vi "test_F9P.vi"() -> ()   [LabVIEW 2019] (continued)
47,33,72,237,38,1*7F\r\n$GBGSV,4,4,13,34,13,141,,1*45\r\n$GBGSV,4,1,13,04,35,133,,05,09,257,,06,27,182,,07,09,201,,3*79\r\n$GBGSV,4,2,13,08,65,355,39,09,07,194,,10,16,222,16,11,38,142,21,3*7C\r\n$GBGSV,4,3,13,13,50,314,29,14,77,038,38,28,58,310,,33,72,237,,3*78\r\n$GBGSV,4,4,13,34,13,141,,3*47\r\n$GNGLL,3723.59889,N,12656.92573,E,064143.00,A,A*7F\r\n$GNRMC,064144.00,A,3723.59887,N,12656.92567,E,0.152,,250720,,,A,V*14\r\n$GNVTG,,T,,M,0.152,N,0.282,K,A*33\r\n$GNGGA,064144.00,3723.59887,N,12656.92567,E,1,12,0.77,63.9,M,18.5,M,,*75\r\n$GNGSA,A,3,17,19,06,05,02,12,09,,,,,,1.38,0.77,1.14,1*0A\r\n$GNGSA,A,3,85,70,71,72,,,,,,,,,1.38,0.77,1.14,2*05\r\n$GNGSA,A,3,36,11,04,09,12,,,,,,,,1.38,0.77,1.14,3*06\r\n$GNGSA,A,3,28,14,13,11,33,08,10,,,,,,1.38,0.77,1.14,4*0E\r\n$GPGSV,4,1,13,02,65,334,43,04,09,037,,05,47,260,41,06,59,075,34,1*60\r\n$GPGSV,4,2,13,07,06,105,,09,39,058,37,12,18,264,29,13,07,191,,1*62\r\n$GPGSV,4,3,13,17,20,157,22,19,38,161,34,25,11,294,,29,06,323,17,1*65\r\n$GPGSV,4,4,13,30,01,134,,1*52\r\n$GPGSV,4,1,13,02,65,334,,04,09,037,,05,47,260,30,06,59,075,21,6*62\r\n$GPGSV,4,2,13,07,06,105,,09,39,058,35,12,18,264,,13,07,191,,6*6C\r\n$GPGSV,4,3,13,17,20,157,,19,38,161,,25,11,294,,29,06,323,,6*63\r\n$GPGSV,4,4,13,30,01,134,,6*55\r\n$GLGSV,2,1,06,70,55,030,33,71,68,223,35,72,17,216,31,84,09,133,10,1*75\r\n$GLGSV,2,2,06,85,63,111,31,86,51,337,,1*78\r\n$GLGSV,2,1,06,70,55,030,,71,68,223,32,72,17,216,22,84,09,133,12,3*70\r\n$GLGSV,2,2,06,85,63,111,35,86,51,337,,3*7E\r\n$GAGSV,3,1,09,02,04,288,08,04,68,087,34,09,44,196,27,11,77,034,37,7*77\r\n$GAGSV,3,2,09,12,32,114,29,18,55,286,45,19,18,042,06,25,01,241,,7*72\r\n$GAGSV,3,3,09,36,34,314,25,7*49\r\n$GAGSV,3,1,09,02,04,288,,04,68,087,33,09,44,196,30,11,77,034,31,2*7D\r\n$GAGSV,3,2,09,12,32,114,15,18,55,286,42,19,18,042,,25,01,241,,2*79\r\n$GAGSV,3,3,09,36,34,314,23,2*4A\r\n$GBGSV,4,1,13,04,35,133,,05,09,257,,06,27,182,,07,09,201,,1*7B\r\n$GBGSV,4,2,13,08,65,355,38,09,07,194,,10,16,222,,11,38,142,24,1*7D\r\n$GBGSV,4,3,13,13,50,314,29,14,77,038,39,28,58,310,46,33,72,237,40,1*7D\r\n$GBGSV,4,4,13,34,13,141,,1*45\r\n$GBGSV,4,1,13,04,35,133,,05,09,257,,06,27,182,,07,09,201,,3*79\r\n$GBGSV,4,2,13,08,65,355,39,09,07,194,,10,16,222,18,11,38,142,33,3*71\r\n$GBGSV,4,3,13,13,50,314,31,14,77,038,38,28,58,310,,33,72,237,,3*71\r\n$GBGSV,4,4,13,34,13,141,,3*47\r\n$GNGLL,3723.59887,N,12656.92567,E,064144.00,A,A*73\r\n$GNRMC,064145.00,A,3723.59896,N,12656.92569,E,0.478,305.82,250720,,,A,V*04\r\n$GNVTG,305.82,T,,M,0.478,N,0.885,K,A*21\r\n$GNGGA,064145.00,3723.59896,N,12656.92569,E,1,12,0.62,63.6,M,18.5,M,,*71\r\n$GNGSA,A,3,17,19,06,05,02,12,09,,,,,,1.08,0.62,0.88,1*09\r\n$GNGSA,A,3,85,70,71,72,,,,,,,,,1.08,0.62,0.88,2*06\r\n$GNGSA,A,3,36,19,11,04,09,12,,,,,,,1.08,0.62,0.88,3*0D\r\n$GNGSA,A,3,28,14,13,11,33,08,10,,,,,,1.08,0.62,0.88,4*0D\r\n$GPGSV,4,1,13,02,65,334,43,04,09,037,24,05,47,260,40,06,59,075,36,1*65\r\n$GPGSV,4,2,13,07,06,105,,09,39,058,39,12,18,264,28,13,07,191,,1*6D\r\n$GPGSV,4,3,13,17,20,157,23,19,38,161,29,25,11,294,,29,06,323,15,1*6A\r\n$GPGSV,4,4,13,30,01,134,,1*52\r\n$GPGSV,4,1,13,02,65,334,,04,09,037,19,05,47,260,35,06,59,075,33,6*6C\r\n$GPGSV,4,2,13,07,06,105,,09,39,058,38,12,18,264,,13,07,191,,6*61\r\n$GPGSV,4,3,13,17,20,157,22,19,38,161,,25,11,294,,29,06,323,,6*63\r\n$GPGSV,4,4,13,30,01,134,,6*55\r\n$GLGSV,2,1,06,70,55,030,28,71,68,223,39,72,17,216,26,84,09,133,10,1*75\r\n$GLGSV,2,2,06,85,63,111,30,86,51,337,,1*79\r\n$GLGSV,2,1,06,70,55,030,,71,68,223,32,72,17,216,22,84,09,133,11,3*73\r\n$GLGSV,2,2,06,85,63,111,30,86,51,337,,3*7B\r\n$GAGSV,3,1,09,02,04,288,08,04,68,087,36,09,44,196,35,11,77,034,39,7*78\r\n$GAGSV,3,2,09,12,32,114,28,18,55,286,47,19,18,042,11,25,01,241,,7*77\r\n$GAGSV,3,3,09,36,34,314,31,7*4C\r\n$GAGSV,3,1,09,02,04,288,,04,68,087,33,09,44,196,29,11,77,034,33,2*77\r\n$GAGSV,3,2,09,12,32,114,19,18,55,286,43,19,18,042,,25,01,241,,2*74\r\n$GAGSV,3,3,09,36,34,314,24,2*4D\r\n$GBGSV,4,1,13,04,35,133,,05,09,257,,06,27,182,,07,09,201,,1*7B\r\n$GBGSV,4,2,13,08,65,355,39,09,07,194,,10,16,222,,11,38,142,22,1*7A\r\n$GBGSV,4,3,13,13,50,314,29,14,77,038,41,28,58,310,44,33,72,237,39,1*7E\r\n$GBGSV,4,4,13,34,13,141,,1*45\r\n$GBGSV,4,1,13,04,35,133,,05,09,257,,06,27,182,,07,09,201,,3*79\r\n$GBGSV,4,2,13,08,65,355,36,09,07,194,,10,16,222,17,11,38,142,31,3*73\r\n$GBGSV,4,3,13,13,50,314,31,14,77,038,35,28,58,310,,33,72,237,,3*7C\r\n$GBGSV,4,4,13,34,13,141,,3*47\r\n$GNGLL,3723.59896,N,12656.92569,E,064145.00,A,A*7C\r\n$GNRMC,064146.00,A,3723.59920,N,12656.92613,E,1.922,48.63,250720,,,A,V*33\r\n$GNVTG,48.63,T,,M,1.922,N,3.560,K,A*12\r\n$GNGGA,064146.00,3723.59920,N,12656.92613,E,1,12,0.65,62.9,M,18.5,M,,*79\r\n$GNGSA,A,3,17,19,06,05,02,12,09,,,,,,1.13,0.65,0.92,1*0F\r\n$GNGSA,A,3,85,70,71,72,,,,,,,,,1.13,0.65,0.92,2*00\r\n$GNGSA,A,3,36,19,11,04,09,12,,,,,,,1.13,0.65,0.92,3*0B\r\n$GNGSA,A,3,28,14,13,11,33,08,10,,,,,,1.13,0.65,0.92,4*0B\r\n$GPGSV,4,1,13,02,65,334,39,04,08,037,22,05,47,260,35,06,59,075,43,1*6F\r\n$GPGSV,4,2,13,07,06,105,,09,39,058,40,12,18,264,20,13,07,191,,1*6B\r\n$GPGSV,4,3,13,17,20,157,22,19,38,161,33,25,11,294,,29,06,323,14,1*61\r\n$GPGSV,4,4,13,30,01,134,,1*52\r\n$GPGSV,4,1,13,02,65,334,,04,08,037,18,05,47,260,34,06,59,075,29,6*66\r\n$GPGSV,4,2,13,07,06,105,,09,39,058,38,12,18,264,23,13,07,191,,6*60\r\n$GPGSV,4,3,13,17,20,157,20,19,38,161,,25,11,294,,29,06,323,,6*61\r\n$GPGSV,4,4,13,30,01,134,,6*55\r\n$GLGSV,2,1,06,70,55,030,28,71,68,223,33,72,17,216,24,84,09,133,08,1*74\r\n$GLGSV,2,2,06,85,63,111,24,86,51,337,,1*7C\r\n$GLGSV,2,1,06,70,55,030,,71,68,223,32,72,17,216,21,84,09,133,09,3*79\r\n$GLGSV,2,2,06,85,63,111,25,86,51,337,,3*7F\r\n$GAGSV,3,1,09,02,04,288,09,04,68,087,32,09,44,196,31,11,77,034,39,7*79\r\n$GAGSV,3,2,09,12,32,114,28,18,55,286,43,19,18,042,16,25,01,241,,7*74\r\n$GAGSV,3,3,09,36,34,314,25,7*49\r\n$GAGSV,3,1,09,02,04,288,,04,68,087,37,09,44,196,29,11,77,034,30,2*70\r\n$GAGSV,3,2,09,12,32,114,25,18,55,286,37,19,18,042,,25,01,241,,2*78\r\n$GAGSV,3,3,09,36,34,314,22,2*4B\r\n$GBGSV,4,1,13,04,35,133,,05,09,257,,06,27,182,,07,09,201,,1*7B\r\n$GBGSV,4,2,13,08,65,355,42,09,07,194,,10,16,222,,11,38,142,23,1*77\r\n$GBGSV,4,3,13,13,50,314,29,14,77,038,42,28,58,310,44,33,72,237,38,1*7C\r\n$GBGSV,4,4,13,34,13,141,,1*45\r\n$GBGSV,4,1,13,04,35,133,,05,09,257,,06,27,182,,07,09,201,,3*79\r\n$GBGSV,4,2,13,08,65,355,36,09,07,194,,10,16,222,18,11,38,142,27,3*7B\r\n$GBGSV,4,3,13,13,50,314,28,14,77,038,34,28,58,310,,33,72,237,,3*75\r\n$GBGSV,4,4,13,34,13,141,,3*47\r\n$GNGLL,3723.59920,N,12656.92613,E,064146.00,A,A*7D\r\n$GNRMC,064147.00,A,3723.59950,N,12656.92680,E,2.195,54.45,250720,,,A,V*31\r\n$GNVTG,54.45,T,,M,2.195,N,4.064,K,A*1A\r\n$GNGGA,064147.00,3723.59950,N,12656.92680,E,1,12,0.67,62.1,M,18.5,M,,*7F\r\n$GNGSA,A,3,17,19,06,05,02,12,09,,,,,,1.15,0.67,0.93,1*0A\r\n$GNGSA,A,3,85,70,71,72,,,,,,,,,1.15,0.67,0.93,2*05\r\n$GNGSA,A,3,36,19,11,04,09,12,,,,,,,1.15,0.67,0.93,3*0E\r\n$GNGSA,A,3,28,14,13,11,33,08,10,,,,,,1.15,0.67,0.93,4*0E\r\n$GPGSV,4,1,13,02,65,334,42,04,08,037,22,05,48,261,29,06,59,075,43,1*60\r\n$GPGSV,4,2,13,07,06,105,,09,39,058,40,12,18,264,21,13,07,191,,1*6A\r\n$GPGSV,4,3,13,17,20,157,22,19,38,161,29,25,11,294,,29,06,323,11,1*6F\r\n$GPGSV,4,4,13,30,01,134,,1*52\r\n$GPGSV,4,1,13,02,65,334,,04,08,037,18,05,48,261,34,06,59,075,40,6*67\r\n$GPGSV,4,2,13,07,06,105,,09,39,058,40,12,18,264,23,13,07,191,,6*6F\r\n$GPGSV,4,3,13,17,20,157,18,19,38,161,,25,11,294,,29,06,323,,6*6A\r\n$GPGSV,4,4,13,30,01,134,,6*55\r\n$GLGSV,2,1,06,70,55,030,28,71,68,223,39,72,17,216,26,84,09,133,08,1*7C\r\n$GLGSV,2,2,06,85,63,111,31,86,51,337,,1*78\r\n$GLGSV,2,1,06,70,55,030,,71,68,223,32,72,17,216,21,84,09,133,13,3*72\r\n$GLGSV,2,2,06,85,63,111,28,86,51,337,,3*72\r\n$GAGSV,3,1,09,02,04,288,09,04,68,087,42,09,44,196,25,11,77,034,39,7*7B\r\n$GAGSV,3,2,09,12,32,114,20,18,55,286,43,19,18,042,20,25,01,241,,7*79\r\n$GAGSV,3,3,09,36,34,314,26,7*4A\r\n$GAGSV,3,1,09,02,04,288,,04,68,087,40,09,44,196,23,11,77,034,31,2*7B\r\n$GAGSV,3,2,09,12,32,114,23,18,55,286,39,19,18,042,,25,01,241,,2*70\r\n$GAGSV,3,3,09,36,34,314,18,2*42\r\n$GBGSV,4,1,13,04,35,133,,05,09,257,,06,27,182,,07,09,201,,1*7B\r\n$GBGSV,4,2,13,08,65,355,38,09,07,194,,10,16,222,,11,38,142,22,1*7B\r\n$GBGSV,4,3,13,13,50,314,23,14,77,038,43,28,58,310,38,33,72,237,40,1*73\r\n$GBGSV,4,4,13,34,13,141,,1*45\r\n$GBGSV,4,1,13,04,35,133,,05,09,257,,06,27,182,,07,09,201,,3*79\r\n$GBGSV,4,2,13,08,65,355,36,09,07,194,,10,16,222,19,11,38,142,27,3*7A\r\n$GBGSV,4,3,13,13,50,314,26,14,77,038,39,28,58,310,,33,72,237,,3*76\r\n$GBGSV,4,4,13,34,13,141,,3*47\r\n$GNGLL,3723.59950,N,12656.92680,E,064147.00,A,A*71\r\n$GNRMC,064148.00,A,3723.59985,N,12656.92753,E,2.416,59.10,250720,,,A,V*3A\r\n$GNVTG,59.10,T,,M,2.416,N,4.474,K,A*1C\r\n$GNGGA,064148.00,3723.59985,N,12656.92753,E,1,12,0.62,61.5,M,18.5,M,,*75\r\n$GNGSA,A,3,17,19,06,05,02,12,09,,,,,,1.08,0.62,0.88,1*09\r\n$GNGSA,A,3,85,70,71,72,,,,,,,,,1.08,0.62,0.88,2*06\r\n$GNGSA,A,3,36,19,11,04,09,12,,,,,,,1.08,0.62,0.88,3*0D\r\n$GNGSA,A,3,28,14,13,11,33,08,10,,,,,,1.08,0.62,0.88,4*0D\r\n$GPGSV,4,1,13,02,65,334,46,04,08,037,21,05,48,261,38,06,58,076,44,1*62\r\n$GPGSV,4,2,13,07,06,105,,09,39,058,41,12,18,264,20,13,07,191,,1*6A\r\n$GPGSV,4,3,13,17,20,157,22,19,38,161,29,25,11,294,,29,06,323,,1*6F\r\n$GPGSV,4,4,13,30,01,134,,1*52\r\n$GPGSV,4,1,13,02,65,334,,04,08,037,29,05,48,261,34,06,58,076,36,6*66\r\n$GPGSV,4,2,13,07,06,105,,09,39,058,42,12,18,264,22,13,07,191,,6*6C\r\n$GPGSV,4,3,13,17,20,157,17,19,38,161,,25,11,294,,29,06,323,,6*65\r\n$GPGSV,4,4,13,30,01,134,,6*55\r\n$GLGSV,2,1,06,70,55,030,34,71,68,223,40,72,17,216,26,84,09,133,09,1*7E\r\n$GLGSV,2,2,06,85,63,111,31,86,51,337,,1*78\r\n$GLGSV,2,1,06,70,55,030,,71,68,223,27,72,17,216,19,84,09,133,08,3*77\r\n$GLGSV,2,2,06,85,63,111,27,86,51,337,,3*7D\r\n$GAGSV,3,1,09,02,04,288,10,04,68,087,42,09,44,196,30,11,77,034,39,7*77\r\n$GAGSV,3,2,09,12,32,114,22,18,55,286,44,19,18,042,20,25,01,241,,7*7C\r\n$GAGSV,3,3,09,36,34,314,25,7*49\r\n$GAGSV,3,1,09,02,04,288,,04,68,087,33,09,44,196,25,11,77,034,32,2*7A\r\n$GAGSV,3,2,09,12,32,114,26,18,55,286,43,19,18,042,,25,01,241,,2*78\r\n$GAGSV,3,3,09,36,34,314,19,2*43\r\n$GBGSV,4,1,13,04,35,133,,05,09,257,,06,27,182,,07,09,201,,1*7B\r\n$GBGSV,4,2,13,08,65,355,42,09,07,194,,10,16,222,,11,38,142,25,1*71\r\n$GBGSV,4,3,13,13,50,314,25,14,77,038,41,28,58,310,31,33,72,237,41,1*7F\r\n$GBGSV,4,4,13,34,13,141,,1*45\r\n$GBGSV,4,1,13,04,35,133,,05,09,257,,06,27,182,,07,09,201,,3*79\r\n$GBGSV,4,2,13,08,65,355,29,09,07,194,,10,16,222,17,11,38,142,27,3*7A\r\n$GBGSV,4,3,13,13,50,314,24,14,77,038,36,28,58,310,,33,72,237,,3*7B\r\n$GBGSV,4,4,13,34,13,141,,3*47\r\n$GNGLL,3723.59985,N,12656.92753,E,064148.00,A,A*79\r\n$GNRMC,064149.00,A,3723.60031,N,12656.92824,E,2.456,54.22,250720,,,A,V*30\r\n$GNVTG,54.22,T,,M,2.456,N,4.548,K,A*1A\r\n$GNGGA,064149.00,3723.60031,N,12656.92824,E,1,12,0.64,60.9,M,18.5,M,,*7C\r\n$GNGSA,A,3,17,19,06,05,02,12,09,,,,,,1.12,0.64,0.92,1*0F\r\n$GNGSA,A,3,85,70,71,72,,,,,,,,,1.12,0.64,0.92,2*00\r\n$GNGSA,A,3,36,19,11,04,09,12,,,,,,,1.12,0.64,0.92,3*0B\r\n$GNGSA,A,3,28,14,13,11,33,08,10,,,,,,1.12,0.64,0.92,4*0B\r\n$GPGSV,4,1,13,02,65,334,46,04,08,037,23,05,48,261,35,06,58,076,45,1*6C\r\n$GPGSV,4,2,13,07,06,105,,09,39,058,41,12,18,264,,13,07,191,,1*68\r\n$GPGSV,4,3,13,17,20,157,22,19,38,161,32,25,11,294,,29,06,323,,1*65\r\n$GPGSV,4,4,13,30,01,134,,1*52\r\n$GPGSV,4,1,13,02,65,334,,04,08,037,32,05,48,261,34,06,58,076,33,6*69\r\n$GPGSV,4,2,13,07,06,105,,09,39,058,42,12,18,264,19,13,07,191,,6*64\r\n$GPGSV,4,3,13,17,20,157,15,19,38,161,,25,11,294,,29,06,323,,6*67\r\n$GPGSV,4,4,13,30,01,134,,6*55\r\n$GLGSV,2,1,06,70,55,030,33,71,68,223,41,72,17,216,26,84,09,133,10,1*70\r\n$GLGSV,2,2,06,85,63,111,38,86,51,337,,1*71\r\n$GLGSV,2,1,06,70,55,030,,71,68,223,29,72,17,216,19,84,09,133,09,3*78\r\n$GLGSV,2,2,06,85,63,111,27,86,51,337,,3*7D\r\n$GAGSV,3,1,09,02,04,288,05,04,68,087,43,09,44,196,29,11,77,034,40,7*74\r\n$GAGSV,3,2,09,12,32,114,22,18,55,286,41,19,18,042,23,25,01,241,,7*7A\r\n$GAGSV,3,3,09,36,34,314,23,7*4F\r\n$GAGSV,3,1,09,02,04,288,,04,68,087,36,09,44,196,24,11,77,034,35,2*79\r\n$GAGSV,3,2,09,12,32,114,25,18,55,286,42,19,18,042,,25,01,241,,2*7A\r\n$GAGSV,3,3,09,36,34,314,17,2*4D\r\n$GBGSV,4,1,13,04,35,133,,05,09,257,,06,27,182,,07,09,201,,1*7B\r\n$GBGSV,4,2,13,08,65,355,42,09,07,194,,10,16,222,19,11,38,142,30,1*7D\r\n$GBGSV,4,3,13,13,50,314,26,14,77,038,44,28,58,310,30,33,72,237,42,1*7B\r\n$GBGSV,4,4,13,34,13,141,,1*45\r\n$GBGSV,4,1,13,04,35,133,,05,09,257,,06,27,182,,07,09,201,,3*79\r\n$GBGSV,4,2,13,08,65,355,30,09,07,194,,10,16,222,19,11,38,142,32,3*78\r\n$GBGSV,4,3,13,13,50,314,22,14,77,038,38,28,58,310,,33,72,237,,3*73\r\n$GBGSV,4,4,13,34,13,141,,3*47\r\n$GNGLL,3723.60031,N,12656.92824,E,064149.00,A,A*7B\r\n$GNRMC,064150.00,A,3723.60070,N,12656.92905,E,2.760,59.14,250720,,,A,V*31\r\n$GNVTG,59.14,T,,M,2.760,N,5.111,K,A*1D\r\n$GNGGA,064150.00,3723.60070,N,12656.92905,E,1,12,0.67,60.4,M,18.5,M,,*7D\r\n$GNGSA,A,3,17,19,06,05,02,12,09,,,,,,1.15,0.67,0.93,1*0A\r\n$GNGSA,A,3,85,70,71,72,,,,,,,,,1.15,0.67,0.93,2*05\r\n$GNGSA,A,3,36,19,11,04,09,12,,,,,,,1.15,0.67,0.93,3*0E\r\n$GNGSA,A,3,28,14,13,11,33,08,10,,,,,,1.15,0.67,0.93,4*0E\r\n$GPGSV,4,1,13,02,65,334,44,04,08,037,25,05,48,261,32,06,58,076,41,1*6B\r\n$GPGSV,4,2,13,07,06,105,,09,39,058,39,12,18,264,24,13,07,191,,1*61\r\n$GPGSV,4,3,13,17,20,157,25,19,38,161,26,25,11,294,,29,06,323,,1*67\r\n$GPGSV,4,4,13,30,01,134,,1*52\r\n$GPGSV,4,1,13,02,65,334,,04,08,037,26,05,48,261,36,06,58,076,36,6*6B\r\n$GPGSV,4,2,13,07,06,105,,09,39,058,40,12,18,264,18,13,07,191,,6*67\r\n$GPGSV,4,3,13,17,20,157,16,19,38,161,,25,11,294,,29,06,323,,6*64\r\n$GPGSV,4,4,13,30,01,134,,6*55\r\n$GLGSV,2,1,06,70,55,030,34,71,68,223,41,72,17,216,32,84,09,133,12,1*70\r\n$GLGSV,2,2,06,85,63,111,38,86,51,337,,1*71\r\n$GLGSV,2,1,06,70,55,030,,71,68,223,28,72,17,216,19,84,09,133,13,3*72\r\n$GLGSV,2,2,06,85,63,111,26,86,51,337,,3*7C\r\n$GAGSV,3,1,09,02,04,288,06,04,68,087,40,09,44,196,28,11,77,034,40,7*75\r\n$GAGSV,3,2,09,12,32,114,24,18,55,286,42,19,18,042,23,25,01,241,,7*7F\r\n$GAGSV,3,3,09,36,34,314,23,7*4F\r\n$GAGSV,3,1,09,02,04,288,,04,68,087,33,09,44,196,24,11,77,034,32,2*7B\r\n$GAGSV,3,2,09,12,32,114,24,18,55,286,43,19,18,042,25,25,01,241,,2*7D\r\n$GAGSV,3,3,09,36,34,314,18,2*42\r\n$GBGSV,4,1,13,04,35,133,,05,09,257,,06,27,182,,07,09,201,,1*7B\r\n$GBGSV,4,2,13,08,65,355,39,09,07,194,,10,16,222,19,11,38,142,33,1*72\r\n$GBGSV,4,3,13,13,50,314,24,14,77,038,44,28,58,310,35,33,72,237,42,1*7C\r\n$GBGSV,4,4,13,34,13,141,,1*45\r\n$GBGSV,4,1,13,04,35,133,,05,09,257,,06,27,182,,07,09,201,,3*79\r\n$GBGSV,4,2,13,08,65,355,33,09,07,194,,10,16,222,19,11,38,142,26,3*7E\r\n$GBGSV,4,3,13,13,50,314,21,14,77,038,36,28,58,310,,33,72,237,,3*7E\r\n$GBGSV,4,4,13,34,13,141,,3*47\r\n$GNGLL,3723.60070,N,12656.92905,E,064150.00,A,A*74\r\n$GNRMC,064151.00,A,3723.60101,N,12656.92993,E,2.794,62.68,250720,,,A,V*30\r\n$GNVTG,62.68,T,,M,2.794,N,5.175,K,A*17\r\n$GNGGA,064151.00,3723.60101,N,12656.92993,E,1,12,0.64,59.7,M,18.5,M,,*7E\r\n$GNGSA,A,3,17,19,06,05,02,12,09,,,,,,1.12,0.64,0.92,1*0F\r\n$GNGSA,A,3,85,70,71,72,,,,,,,,,1.12,0.64,0.92,2*00\r\n$GNGSA,A,3,36,19,11,04,09,12,,,,,,,1.12,0.64,0.92,3*0B\r\n$GNGSA,A,3,28,14,13,11,33,08,10,,,,,,1.12,0.64,0.92,4*0B\r\n$GPGSV,4,1,13,02,65,334,45,04,08,037,24,05,48,261,38,06,58,076,41,1*61\r\n$GPGSV,4,2,13,07,06,105,,09,38,057,38,12,18,264,26,13,07,191,,1*6C\r\n$GPGSV,4,3,13,17,20,157,25,19,38,161,27,25,11,294,,29,06,323,,1*66\r\n$GPGSV,4,4,13,30,01,134,,1*52\r\n$GPGSV,4,1,13,02,65,334,,04,08,037,25,05,48,261,36,06,58,076,30,6*6E\r\n$GPGSV,4,2,13,07,06,105,,09,38,057,41,12,18,264,16,13,07,191,,6*66\r\n$GPGSV,4,3,13,17,20,157,20,19,38,161,,25,11,294,,29,06,323,,6*61\r\n$GPGSV,4,4,13,30,01,134,,6*55\r\n$GLGSV,2,1,06,70,55,030,30,71,68,223,37,72,17,216,27,84,09,133,12,1*71\r\n$GLGSV,2,2,06,85,63,111,30,86,51,337,,1*79\r\n$GLGSV,2,1,06,70,55,030,,71,68,223,28,72,17,216,18,84,09,133,06,3*77\r\n$GLGSV,2,2,06,85,63,111,26,86,51,337,,3*7C\r\n$GAGSV,3,1,09,02,04,288,08,04,68,087,40,09,44,196,27,11,77,034,38,7*7B\r\n$GAGSV,3,2,09,12,32,114,26,18,55,286,39,19,18,042,24,25,01,241,,7*76\r\n$GAGSV,3,3,09,36,34,314,24,7*48\r\n$GAGSV,3,1,09,02,04,288,,04,68,087,31,09,44,196,25,11,77,034,33,2*79\r\n$GAGSV,3,2,09,12,32,114,24,18,55,286,38,19,18,042,25,25,01,241,,2*71\r\n$GAGSV,3,3,09,36,34,314,18,2*42\r\n$GBGSV,4,1,13,04,35,133,,05,09,257,,06,27,182,,07,09,201,,1*7B\r\n$GBGSV,4,2,13,08,65,355,41,09,07,194,,10,16,222,18,11,38,142,29,1*77\r\n$GBGSV,4,3,13,13,50,314,23,14,77,038,43,28,58,310,36,33,72,237,39,1*73\r\n$GBGSV,4,4,13,34,13,141,,1*45\r\n$GBGSV,4,1,13,04,35,133,,05,09,257,,06,27,182,,07,09,201,,3*79\r\n$GBGSV,4,2,13,08,65,355,28,09,07,194,,10,16,222,20,11,38,142,33,3*7A\r\n$GBGSV,4,3,13,13,50,314,20,14,77,038,41,28,58,310,,33,72,237,,3*7F\r\n$GBGSV,4,4,13,34,13,141,,3*47\r\n$GNGLL,3723.60101,N,12656.92993,E,064151.00,A,A*7D\r\n$GNRMC,064152.00,A,3723.60133,N,12656.93077,E,2.709,65.19,250720,,,A,V*35\r\n$GNVTG,65.19,T,,M,2.709,N,5.018,K,A*18\r\n$GNGGA,064152.00,3723.60133,N,12656.93077,E,1,12,0.64,59.2,M,18.5,M,,*7B\r\n$GNGSA,A,3,17,19,06,05,02,12,09,,,,,,1.12,0.64,0.92,1*0F\r\n$GNGSA,A,3,85,70,71,72,,,,,,,,,1.12,0.64,0.92,2*00\r\n$GNGSA,A,3,36,19,11,04,09,12,,,,,,,1.12,0.64,0.92,3*0B\r\n$GNGSA,A,3,28,14,13,11,33,08,10,,,,,,1.12,0.64,0.92,4*0B\r\n$GPGSV,4,1,13,02,65,334,42,04,08,037,25,05,48,261,41,06,58,076,45,1*6D\r\n$GPGSV,4,2,13,07,06,105,,09,38,057,39,12,18,264,24,13,07,191,,1*6F\r\n$GPGSV,4,3,13,17,20,157,25,19,38,161,26,25,11,294,,29,06,323,,1*67\r\n$GPGSV,4,4,13,30,01,134,,1*52\r\n$GPGSV,4,1,13,02,65,334,,04,08,037,22,05,48,261,35,06,58,076,35,6*6F\r\n$GPGSV,4,2,13,07,06,105,,09,38,057,41,12,18,264,18,13,07,191,,6*68\r\n$GPGSV,4,3,13,17,20,157,20,19,38,161,,25,11,294,,29,06,323,,6*61\r\n$GPGSV,4,4,13,30,01,134,,6*55\r\n$GLGSV,2,1,06,70,55,030,30,71,68,223,41,72,17,216,27,84,09,133,09,1*7A\r\n$GLGSV,2,2,06,85,63,111,30,86,51,337,,1*79\r\n$GLGSV,2,1,06,70,55,030,,71,68,223,27,72,17,216,18,84,09,133,06,3*78\r\n$GLGSV,2,2,06,85,63,111,26,86,51,337,,3*7C\r\n$GAGSV,3,1,09,02,04,288,10,04,68,087,38,09,44,196,27,11,77,034,36,7*73\r\n$GAGSV,3,2,09,12,32,114,32,18,55,286,39,19,18,042,24,25,01,241,,7*73\r\n$GAGSV,3,3,09,36,34,314,24,7*48\r\n$GAGSV,3,1,09,02,04,288,,04,68,087,32,09,44,196,25,11,77,034,33,2*7A\r\n$GAGSV,3,2,09,12,32,114,30,18,55,286,42,19,18,042,26,25,01,241,,2*7A\r\n$GAGSV,3,3,09,36,34,314,19,2*43\r\n$GBGSV,4,1,13,04,35,133,,05,09,257,,06,27,182,,07,09,201,,1*7B\r\n$GBGSV,4,2,13,08,65,355,42,09,07,194,,10,16,222,19,11,38,142,34,1*79\r\n$GBGSV,4,3,13,13,50,314,24,14,77,038,40,28,58,310,37,33,72,237,40,1*78\r\n$GBGSV,4,4,13,34,13,141,,1*45\r\n$GBGSV,4,1,13,04,35,133,,05,09,257,,06,27,182,,07,09,201,,3*79\r\n$GBGSV,4,2,13,08,65,355,33,09,07,194,,10,16,222,20,11,38,142,36,3*75\r\n$GBGSV,4,3,13,13,50,314,20,14,77,038,40,28,58,310,,33,72,237,,3*7E\r\n$GBGSV,4,4,13,34,13,141,,3*47\r\n$GNGLL,3723.60133,N,12656.93077,E,064152.00,A,A*7D\r\n$GNRMC,064153.00,A,3723.60163,N,12656.93152,E,2.294,64.02,250720,,,A,V*3D\r\n$GNVTG,64.02,T,,M,2.294,N,4.248,K,A*14\r\n$GNGGA,064153.00,3723.60163,N,12656.93152,E,1,12,0.64,58.5,M,18.5,M,,*7F\r\n$GNGSA,A,3,17,19,06,05,02,12,09,,,,,,1.12,0.64,0.92,1*0F\r\n$GNGSA,A,3,85,70,71,72,,,,,,,,,1.12,0.64,0.92,2*00\r\n$GNGSA,A,3,36,19,11,04,09,12,,,,,,,1.12,0.64,0.92,3*0B\r\n$GNGSA,A,3,28,14,13,11,33,08,10,,,,,,1.12,0.64,0.92,4*0B\r\n$GPGSV,4,1,13,02,65,334,43,04,08,037,26,05,48,261,34,06,58,076,46,1*6E\r\n$GPGSV,4,2,13,07,06,105,,09,38,057,44,12,18,264,24,13,07,191,,1*65\r\n$GPGSV,4,3,13,17,20,157,26,19,38,161,26,25,11,294,,29,06,323,,1*64\r\n$GPGSV,4,4,13,30,01,134,,1*52\r\n$GPGSV,4,1,13,02,65,334,,04,08,037,20,05,48,261,37,06,58,076,32,6*68\r\n$GPGSV,4,2,13,07,06,105,,09,38,057,43,12,18,264,18,13,07,191,,6*6A\r\n$GPGSV,4,3,13,17,20,157,20,19,38,161,,25,11,294,,29,06,323,,6*61\r\n$GPGSV,4,4,13,30,01,134,,6*55\r\n$GLGSV,2,1,06,70,55,030,31,71,68,223,35,72,17,216,27,84,09,133,11,1*71\r\n$GLGSV,2,2,06,85,63,111,30,86,51,337,,1*79\r\n$GLGSV,2,1,06,70,55,030,,71,68,223,27,72,17,216,18,84,09,133,07,3*79\r\n$GLGSV,2,2,06,85,63,111,27,86,51,337,,3*7D\r\n$GAGSV,3,1,09,02,04,288,11,04,68
